vi "Actor Core.vi"(8 "error in":errorcluster, 11 "MainView in":refnum<class "MainView.lvclass">) -> (0 "error out":errorcluster, 3 "Actor out":refnum<class "Actor.lvclass">)   [LabVIEW 2012, in "Win8uiFramework.lvlib" / "MainView.lvclass"]
doc: "(<B>Filename</B>: Actor Framework.lvlib:Actor.lvclass:Actor Core.vi)\n\nReceives messages to the actor, reacts to them, and initiates any error handling that may shut the actor down.\n\nDescendant classes may override this VI to append parallel tasks for the actor to complete while it handles messages. Overrides use the Call Parent Method node."
uses:
  MainView.lvclass
  <vilib>/ActorFramework/Actor/Actor.lvclass
  ViewableActor.lvclass
panel:
  out "Color Box":u32(colorbox)
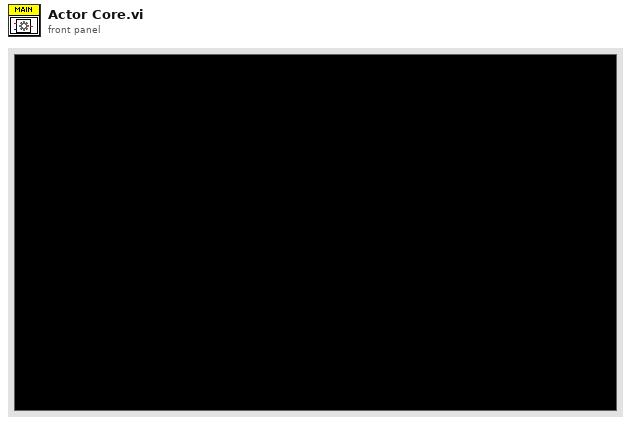
[diagram p1: front panel]
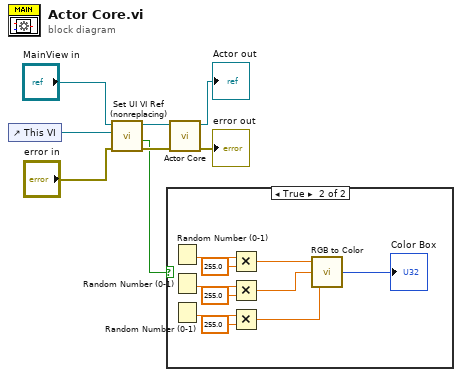
[diagram p0: block diagram]
diagram:
  n1 = control-ref of="This VI"() -> (w3:refnum<vi>)
  n2 = call "Set UI VI Ref (nonreplacing).vi"("error in (no error)"="error in", "UI VI Ref"=w3, "ViewableActor in"="MainView in") -> ("error out"=w5:errorcluster, "Top Level UI?"=w1:bool, "ViewableActor out"=w6:refnum<class "MainView.lvclass">)  [unwired: 6 in]
  n3 = case shown="True" w1 {
    frame False {
    }
    frame True {
      n4 = Random Number (0-1)() -> (number: 0 to 1=w18:dbl)
      n5 = Random Number (0-1)() -> (number: 0 to 1=w13:dbl)
      n6 = Random Number (0-1)() -> (number: 0 to 1=w12:dbl)
      n7 = Multiply(x=w18, y=255.0) -> (x*y=w15:dbl)
      n8 = Multiply(x=w13, y=255.0) -> (x*y=w10:dbl)
      n9 = Multiply(x=w12, y=255.0) -> (x*y=w9:dbl)
      n10 = call <vilib>:"RGB to Color.vi"("B"=w9, "G"=w10, "R"=w15) -> ("Color"=→"Color Box":u32)
    }
  }
  n11 = call-parent "Actor Core.vi"("error in"=w5, "Actor in"=w6) -> ("error out"=→"error out":errorcluster, "Actor out"=→"Actor out":refnum<class "Actor.lvclass">)  [unwired: 8 in]
